vi "GEA3 Flow Stop Algorithim.vi"(0 "Input":T1, 1 "ERD Data":T2, 5 "error in (no error)":errorcluster) -> (14 "Output":T1, 19 "error out":errorcluster)   [LabVIEW 2016]
uses:
  Type Definitions/GEA3 HEWH ERD Data.ctl
  Type Definitions/GEA3 HEWH Mixing Valve.ctl
  type defs/EMV Flow Stop Detection.ctl
panel:
  out "MixValveAbsoluteStepPosition (0x400B)":i16
  out "Position End of Flow?":bool
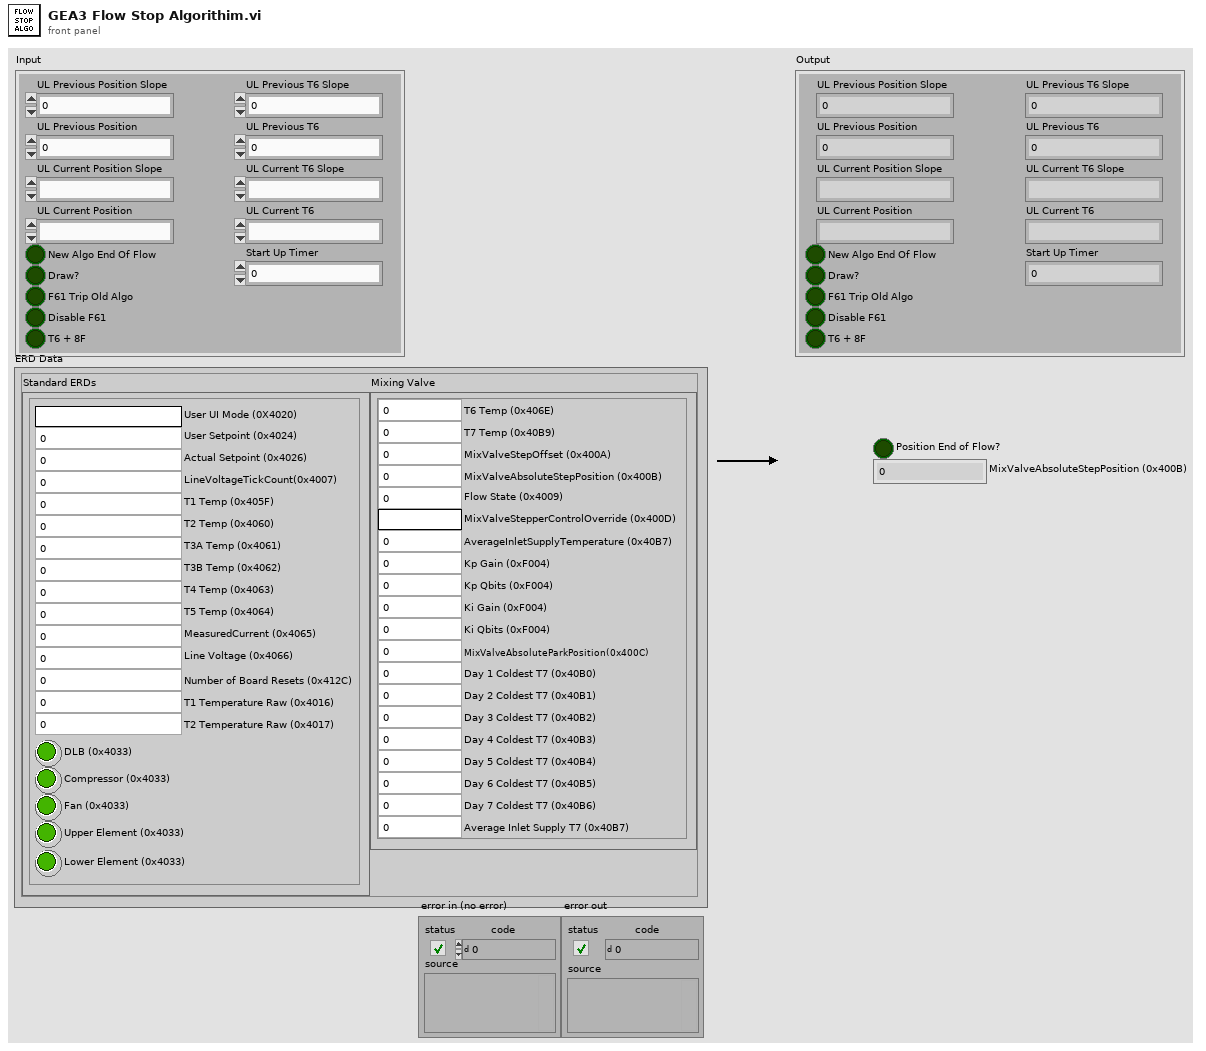
[diagram p1: front panel]
types:
  T1 = typedef "EMV Flow Stop Detection.ctl" = cluster{"UL Previous Position Slope":dbl, "UL Previous T6 Slope":dbl, "UL Previous Position":dbl, "UL Previous T6":dbl, "UL Current Position":dbl, "UL Current Position Slope":dbl, "UL Current T6":dbl, "UL Current T6 Slope":dbl, "New Algo End Of Flow":bool, "Start Up Timer":dbl, "Draw?":bool, "Disable F61":bool, "F61 Trip Old Algo":bool, "T6 + 8F":bool}
  T2 = typedef "GEA3 HEWH ERD Data.ctl" = cluster{"Mixing Valve":T3, "Standard ERDs":cluster{"User UI Mode (0X4020)":string, "User Setpoint (0x4024)":u16, "Actual Setpoint (0x4026)":u16, "DLB (0x4033)":bool, "Compressor (0x4033)":bool, "Lower Element (0x4033)":bool, "Upper Element (0x4033)":bool, "Fan (0x4033)":bool, "T1 Temp (0x405F)":dbl, "T2 Temp (0x4060)":dbl, "T3A Temp (0x4061)":dbl, "T3B Temp (0x4062)":dbl, "T4 Temp (0x4063)":dbl, "T5 Temp (0x4064)":dbl, "Line Voltage (0x4066)":dbl, "MeasuredCurrent (0x4065)":dbl, "LineVoltageTickCount(0x4007)":u16, "Number of Board Resets (0x412C)":u16, "T1 Temperature Raw (0x4016)":u16, "T2 Temperature Raw (0x4017)":u16}}
  T3 = typedef "GEA3 HEWH Mixing Valve.ctl" = cluster{"T7 Temp (0x40B9)":dbl, "MixValveStepOffset (0x400A)":i16, "MixValveAbsoluteStepPosition (0x400B)":i16, "Flow State (0x4009)":u8, "MixValveStepperControlOverride (0x400D)":string, "AverageInletSupplyTemperature (0x40B7)":dbl, "T6 Temp (0x406E)":dbl, "Kp Gain (0xF004)":u16, "Kp Qbits (0xF004)":u16, "Ki Gain (0xF004)":u16, "Ki Qbits (0xF004)":u16, "MixValveAbsoluteParkPosition(0x400C)":i16, "Day 2 Coldest T7 (0x40B1)":dbl, "Day 1 Coldest T7 (0x40B0)":dbl, "Day 4 Coldest T7 (0x40B3)":dbl, "Day 3 Coldest T7 (0x40B2)":dbl, "Day 6 Coldest T7 (0x40B5)":dbl, "Day 5 Coldest T7 (0x40B4)":dbl, "Average Inlet Supply T7 (0x40B7)":dbl, "Day 7 Coldest T7 (0x40B6)":dbl}
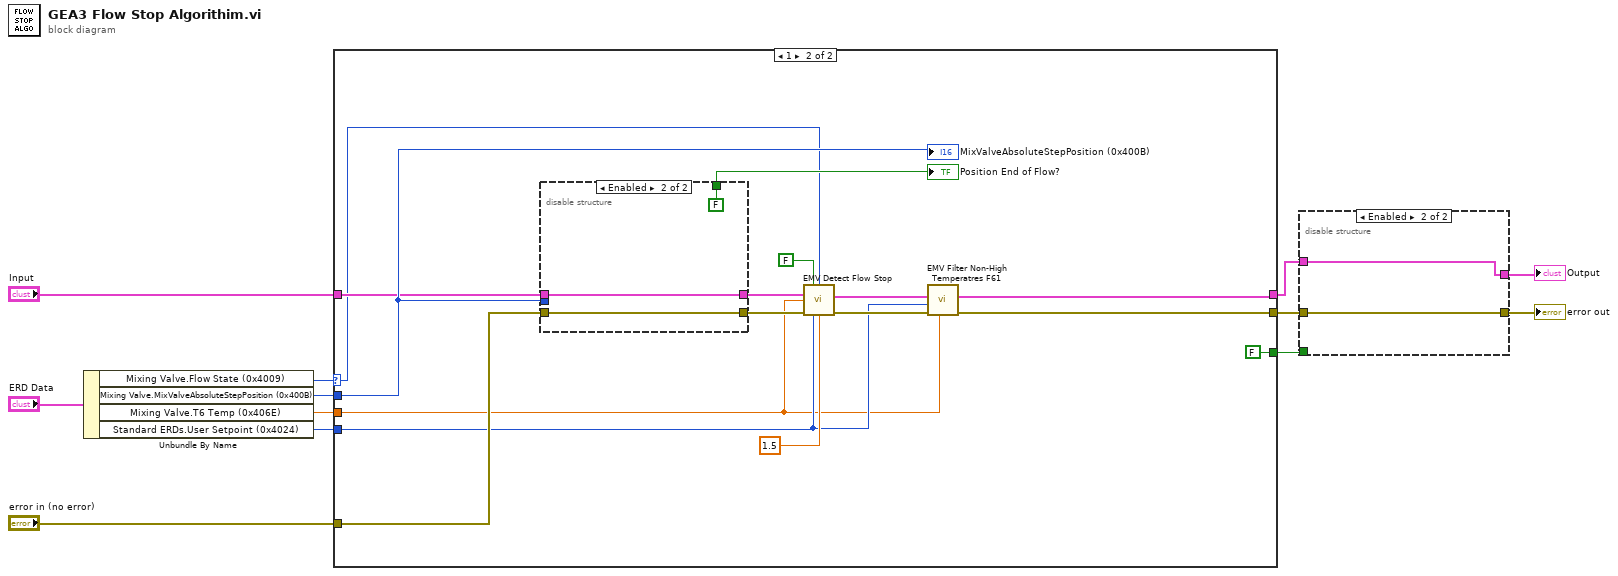
[diagram p0: block diagram]
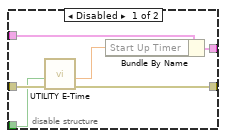
[diagram p2: hidden frame]
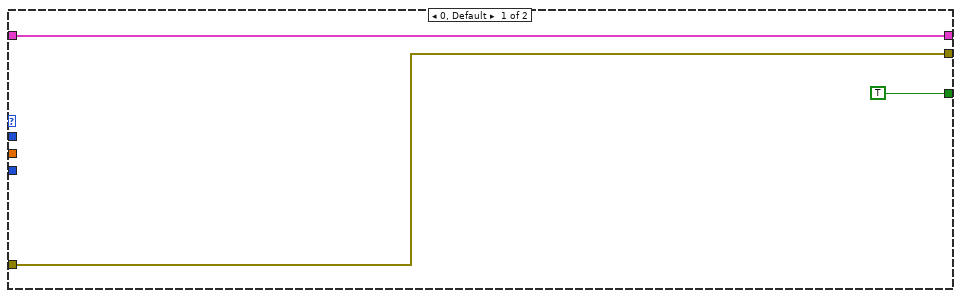
[diagram p3: hidden frame]
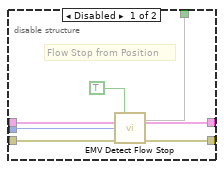
[diagram p4: hidden frame]
diagram:
  n1 = Unbundle By Name("ERD Data") -> ("Mixing Valve.Flow State (0x4009)"=w8:u8, "Mixing Valve.MixValveAbsoluteStepPosition (0x400B)"=w1:i16, "Mixing Valve.T6 Temp (0x406E)"=w12:dbl, "Standard ERDs.User Setpoint (0x4024)"=w9:u16)
  n2 = case shown="1" w8 {
    selector: w8 -> [_ w23]
    tunnel: w12 -> [_ w16]
    tunnel: w1 -> [_ w29]
    tunnel: [w15 w20] -> w6
    tunnel: "error in (no error)" -> [w15 w30]
    tunnel: w9 -> [_ w19]
    tunnel: "Input" -> [w14 w27]
    tunnel: [w14 w17] -> w3
    tunnel: [TRUE FALSE] -> w4
    frame 0, Default {
    }
    frame 1 {
      n3 = disable-structure shown="Enabled" {
        disable-tunnel: [w38 w40] -> w31
        disable-tunnel: w30 -> [w37 w40]
        disable-tunnel: w29 -> [w36 _]
        disable-tunnel: [w35 FALSE ("Position End of Flow?")] -> w28
        disable-tunnel: w27 -> [w34 w41]
        disable-tunnel: [w33 w41] -> w26
        frame Disabled {
          # "Flow Stop from Position"
          n4 = call "EMV Detect Flow Stop.vi"("Position?"=TRUE, "Input"=w34, "T6"=w36, "error in (no error)"=w37) -> ("Output"=w33:T1, 8:w35, "error out"=w38:errorcluster)  [unwired: 8 in, 1 out]
        }
        frame Enabled {
        }
      }
      "Position End of Flow?" <- w28
      n5 = call "EMV Detect Flow Stop.vi"("Position?"=FALSE, "Flow State (0x4009)"=w23, "Input"=w26, "T6"=w16, "error in (no error)"=w31, "User Setpoint (0x4024)"=w19, "Est. Temp Rise"=1.5) -> ("Output"=w18:T1, "error out"=w21:errorcluster)  [unwired: 6 in, 1 out]
      n6 = call "EMV Filter Non-High Temperatres F61.vi"("T6 Temperature"=w16, "error in (no error)"=w21, "User Setpoint (0x4024) in"=w19, "Output in"=w18) -> ("error out"=w20:errorcluster, "Output out"=w17:T1)  [unwired: 6 in]
      "MixValveAbsoluteStepPosition (0x400B)" <- w29
    }
  }
  n7 = disable-structure shown="Enabled" {
    disable-tunnel: w6 -> [w47 w49]
    disable-tunnel: [w46 w49] -> w5
    disable-tunnel: w4 -> [w45 _]
    disable-tunnel: w3 -> [w44 w48]
    disable-tunnel: [w43 w48] -> w2
    frame Disabled {
      n8 = call "UTILITY E-Time.vi"("error in (no error)"=w47, "Reset"=w45) -> ("error out"=w46:errorcluster, "Elapsed Time (sec)"=w42:dbl)  [unwired: 7 in, 1 out]
      n9 = Bundle By Name(cluster=w44, "Start Up Timer"=w42) -> (w43:T1)
    }
    frame Enabled {
    }
  }
  "error out" <- w5
  "Output" <- w2
